vi "Add Protection.vi"(8 "error in (no error)":errorcluster, 9 "Pad":bool, 10 "String in":string, 11 "Checksum U8 in":refnum<class "Checksum U8.lvclass">) -> (0 "error out":errorcluster, 2 "String out":string, 3 "Checksum U8 out":refnum<class "Checksum U8.lvclass">)   [LabVIEW 2013, in "Protections.lvlib" / "Checksum U8.lvclass"]
uses:
  Checksum U8.lvclass
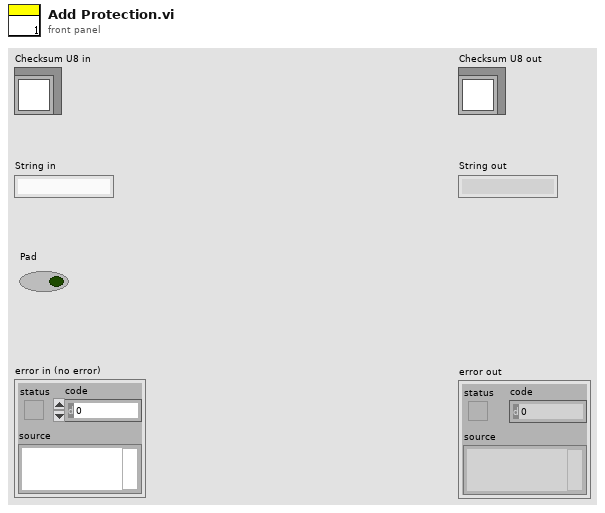
[diagram p1: front panel]
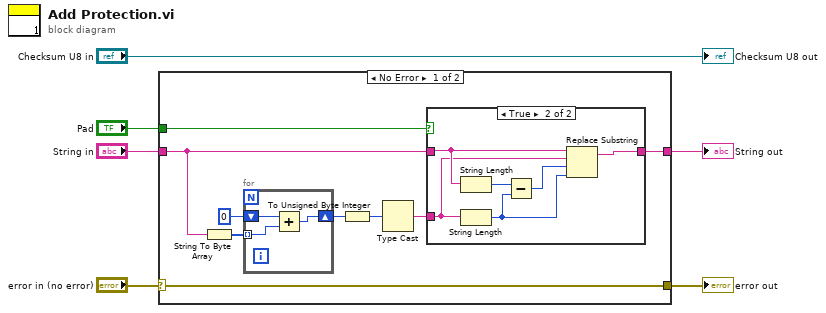
[diagram p0: block diagram]
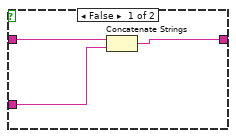
[diagram p2: hidden frame]
diagram:
  n1 = case shown="No Error" "error in (no error)" {
    selector: "error in (no error)" -> [w7 w29]
    tunnel: "Pad" -> [w15 _]
    tunnel: "String in" -> [w14 w28]
    tunnel: [w8 w28] -> w3
    tunnel: [w7 w29] -> w1
    frame No Error {
      n2 = String To Byte Array(string=w14) -> (unsigned byte array=w13:u8[])
      n3 = for {
        tunnel: w13 -> [w27] mode=indexing
        shift-right: [w25] -> w11
        shift-left: u64 0 -> [w26]
        n4 = Add(x=w26, y=w27) -> (x+y=w25:u64)
      }
      n5 = To Unsigned Byte Integer(number=w11) -> (unsigned 8bit integer=w9:u8)
      n6 = Type Cast(x=w9) -> (*(type *) &x=w10:string)  [unwired: 1 in]
      n7 = case shown="True" w15 {
        tunnel: w10 -> [w18 w19]
        tunnel: w14 -> [w17 w23]
        tunnel: [w16 w24] -> w8
        frame False {
          n8 = Concatenate Strings(w17, w18) -> (w16:string)
        }
        frame True {
          n9 = String Length(string=w23) -> (length=w22:i32)
          n10 = String Length(string=w19) -> (length=w21:i32)
          n11 = Subtract(x=w22, y=w21) -> (x-y=w20:i32)
          n12 = Replace Substring(2:w21, 3:w20, 4:w19, 5:w23) -> (1:w24:string)  [unwired: 1 out]
        }
      }
    }
    frame Error {
    }
  }
  "error out" <- w1
  "String out" <- w3
  "Checksum U8 out" <- "Checksum U8 in"
